vi "KE622x -- Delta Mode Set Params.vi"(0 "Resource In":refnum<visa-resource-name>, 1 "Check For SCPI Errors? (T)":bool=TRUE, 7 "Delta Mode Params In":T1={"High Level (A)"=0.001, "Low Level (A)"=-0.001, "Delay (s)"=0.002, "Num Cycles Mode"=enum."Finite Count", "Finite Count"=1, "Abort On\nCompliance?"=FALSE, "Cold Swithing\nMode Enabled?"=FALSE} {"Finite Count" min=1 max=65536; "Low Level (A)" min=-0.105 max=0.0 format="%.3p"; "High Level (A)" min=0.0 max=0.105 format="%.3p"; "Delay (s)" min=0.001 max=9999.999 format="%.3f"}, 11 "error in (no error)":errorcluster, 12 "Read Back Set Values? (T)":bool=TRUE) -> (4 "Resource Out (dupl)":refnum<visa-resource-name>, 8 "Delta Mode Params Out":T1={"High Level (A)"=0.001, "Low Level (A)"=-0.001, "Delay (s)"=0.002, "Num Cycles Mode"=enum."Finite Count", "Finite Count"=1, "Abort On\nCompliance?"=FALSE, "Cold Swithing\nMode Enabled?"=FALSE} {"Finite Count" min=1 max=65536; "Low Level (A)" min=-0.105 max=0.0 format="%.3p"; "High Level (A)" min=0.0 max=0.105 format="%.3p"; "Delay (s)" min=0.001 max=9999.999 format="%.3f"}, 15 "error out":errorcluster)   [LabVIEW 2019, in "Keithley 622x.lvlib"]
doc: "Sets the parameters for 'Delta' measurements. Note that performing this measurement implies that the 622x is being used in conjuction with a 2182/2182A nano-voltmeter."
uses:
  Keithley 622x.lvlib
  Typedefs/KE622x -- Delta Mode Params.ctl
  Low Level/Typedefs/KE622x -- Delta PDelta Mode High Level.ctl
  Low Level/Typedefs/KE622x -- Delta PDelta Mode Low Level.ctl
  Low Level/Typedefs/KE622x -- Delta DCon Mode Delay.ctl
  Low Level/Typedefs/KE622x -- Delta PDelta Mode Num Cycles Mode.ctl
  Low Level/Typedefs/KE622x -- Delta PDelta Mode Num Cycles.ctl
  Trace Buf/Low Level/Typedefs/KE622x -- Trace Buf Size.ctl
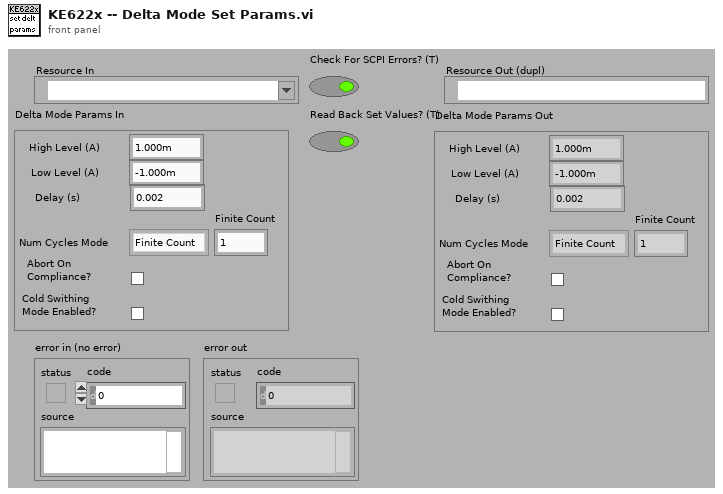
[diagram p1: front panel]
types:
  T1 = typedef "Keithley 622x.lvlib/KE622x -- Delta Mode Params.ctl" = cluster{"High Level (A)":T2, "Low Level (A)":T3, "Delay (s)":T4, "Num Cycles Mode":T5, "Finite Count":T6, "Abort On\nCompliance?":bool, "Cold Swithing\nMode Enabled?":bool}
  T2 = typedef "Keithley 622x.lvlib/KE622x -- Delta PDelta Mode High Level.ctl" = dbl
  T3 = typedef "Keithley 622x.lvlib/KE622x -- Delta PDelta Mode Low Level.ctl" = dbl
  T4 = typedef "Keithley 622x.lvlib/KE622x -- Delta DCon Mode Delay.ctl" = dbl
  T5 = typedef "Keithley 622x.lvlib/KE622x -- Delta PDelta Mode Num Cycles Mode.ctl" = enum16{"Finite Count", "Infinite"}
  T6 = typedef "Keithley 622x.lvlib/KE622x -- Delta PDelta Mode Num Cycles.ctl" = u32
  T7 = typedef "Keithley 622x.lvlib/KE622x -- Trace Buf Size.ctl" = u32
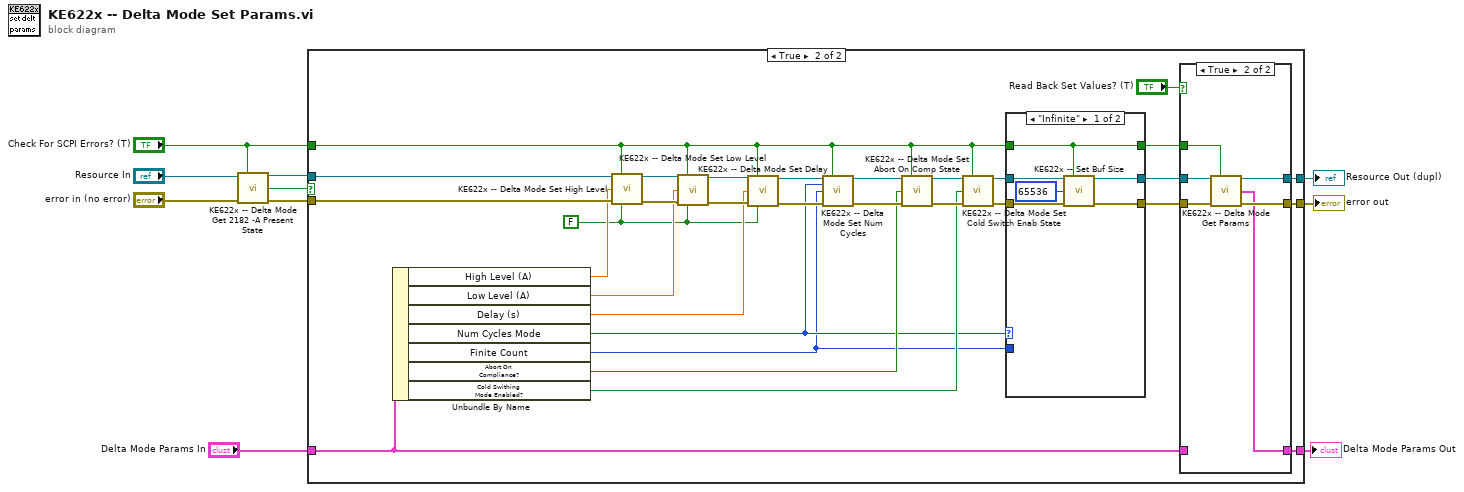
[diagram p0: block diagram]
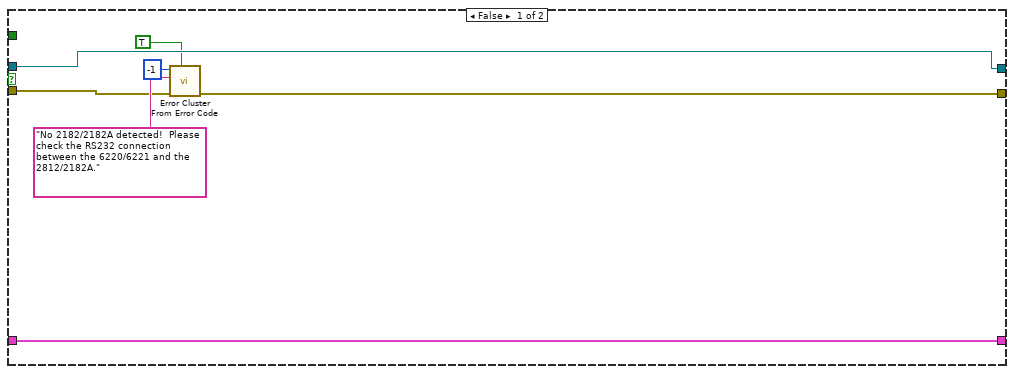
[diagram p2: hidden frame]
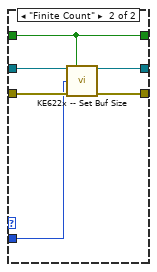
[diagram p3: hidden frame]
diagram:
  n1 = call "KE622x -- Delta Mode Get 2182 -A Present State.vi"("Resource In"="Resource In", "Check For SCPI Errors? (T)"="Check For SCPI Errors? (T)", "error in (no error)"="error in (no error)") -> ("Resource Out (dupl)"=w4:refnum<visa-resource-name>, "2182/2182A Present?"=w2:bool, "error out"=w3:errorcluster)  [unwired: 10 in]
  n2 = case shown="True" w2 {
    tunnel: w4 -> [w13 w48]
    tunnel: w3 -> [w15 w47]
    tunnel: [w13 w29] -> w10
    tunnel: [w14 w28] -> w9
    tunnel: "Delta Mode Params In" -> [w12 w27]
    tunnel: [w12 w26] -> w7
    tunnel: "Check For SCPI Errors? (T)" -> [_ w19]
    frame False {
      n3 = call <vilib>:"Error Cluster From Error Code.vi"("show call chain? (False)"=TRUE, "error in (no error)"=w15, "error message (\"\")"="No 2182/2182A detected!  Please check the RS232 connection between the 6220/6221 and the 2812/2182A.", "error code (0)"=-1) -> ("error out"=w14:errorcluster)  [unwired: 5 in]
    }
    frame True {
      w31 = FALSE ("Read Back Set Value? (T)")
      n4 = Unbundle By Name(w27) -> ("High Level (A)"=w36:T2, "Low Level (A)"=w35:T3, "Delay (s)"=w34:T4, "Num Cycles Mode"=w25:T5, "Finite Count"=w22:T6, "Abort On\nCompliance?"=w33:bool, "Cold Swithing\nMode Enabled?"=w32:bool)
      n5 = call "KE622x -- Delta Mode Set High Level.vi"("Resource In"=w48, "Check For SCPI Errors? (T)"=w19, "High Level In (A)"=w36, "error in (no error)"=w47, "Read Back Set Value? (T)"=w31) -> ("Resource Out (dupl)"=w46:refnum<visa-resource-name>, "error out"=w45:errorcluster)  [unwired: 8 in, 1 out]
      n6 = call "KE622x -- Delta Mode Set Low Level.vi"("Resource In"=w46, "Check For SCPI Errors? (T)"=w19, "Low Level In (A)"=w35, "error in (no error)"=w45, "Read Back Set Value? (T)"=w31) -> ("Resource Out (dupl)"=w44:refnum<visa-resource-name>, "error out"=w43:errorcluster)  [unwired: 8 in, 1 out]
      n7 = call "KE622x -- Delta Mode Set Delay.vi"("Resource In"=w44, "Check For SCPI Errors? (T)"=w19, "Delay In (s)"=w34, "error in (no error)"=w43, "Read Back Set Value? (T)"=w31) -> ("Resource Out (dupl)"=w42:refnum<visa-resource-name>, "error out"=w41:errorcluster)  [unwired: 8 in, 1 out]
      n8 = call "KE622x -- Delta Mode Set Num Cycles.vi"("Resource In"=w42, "Check For SCPI Errors? (T)"=w19, "Num Cycles Mode"=w25, "Num Cycles"=w22, "error in (no error)"=w41) -> ("Resource Out (dupl)"=w38:refnum<visa-resource-name>, "error out"=w37:errorcluster)  [unwired: 9 in]
      n9 = call "KE622x -- Delta Mode Set Abort On Comp State.vi"("Resource In"=w38, "Check For SCPI Errors? (T)"=w19, "Abort On Compliance?"=w33, "error in (no error)"=w37) -> ("Resource Out (dupl)"=w40:refnum<visa-resource-name>, "error out"=w39:errorcluster)  [unwired: 10 in]
      n10 = call "KE622x -- Delta Mode Set Cold Switch Enab State.vi"("Resource In"=w40, "Check For SCPI Errors? (T)"=w19, "Enable Cold Switching Mode?"=w32, "error in (no error)"=w39) -> ("Resource Out (dupl)"=w24:refnum<visa-resource-name>, "error out"=w23:errorcluster)  [unwired: 10 in]
      n11 = case shown="\"Infinite\"" w25 {
        tunnel: w24 -> [w54 w60]
        tunnel: w23 -> [w53 w59]
        tunnel: w22 -> [_ w56]
        tunnel: [w51 w58] -> w21
        tunnel: [w50 w57] -> w20
        tunnel: w19 -> [w49 w55]
        tunnel: [w49 w55] -> w18
        frame "Infinite" {
          n12 = call "KE622x -- Set Buf Size.vi"("Resource In"=w54, "Check For SCPI Errors? (T)"=w49, "Buffer Size (Num Readings)"=T7 65536, "error in (no error)"=w53) -> ("Resource Out (dupl)"=w51:refnum<visa-resource-name>, "error out"=w50:errorcluster)  [unwired: 10 in]
        }
        frame "Finite Count" {
          n13 = call "KE622x -- Set Buf Size.vi"("Resource In"=w60, "Check For SCPI Errors? (T)"=w55, "Buffer Size (Num Readings)"=w56, "error in (no error)"=w59) -> ("Resource Out (dupl)"=w58:refnum<visa-resource-name>, "error out"=w57:errorcluster)  [unwired: 10 in]
        }
      }
      n14 = case shown="True" "Read Back Set Values? (T)" {
        tunnel: w21 -> [w63 w69]
        tunnel: w20 -> [w62 w68]
        tunnel: [w63 w67] -> w29
        tunnel: [w62 w66] -> w28
        tunnel: w27 -> [w61 _]
        tunnel: [w61 w65] -> w26
        tunnel: w18 -> [_ w64]
        frame False {
        }
        frame True {
          n15 = call "KE622x -- Delta Mode Get Params.vi"("Resource In"=w69, "Check For SCPI Errors? (T)"=w64, "error in (no error)"=w68) -> ("Resource Out (dupl)"=w67:refnum<visa-resource-name>, "Delta Mode Params"=w65:T1, "error out"=w66:errorcluster)  [unwired: 10 in]
        }
      }
    }
  }
  "Resource Out (dupl)" <- w10
  "error out" <- w9
  "Delta Mode Params Out" <- w7
